vi "configure filter.vi"(7 "extended id? (F)":bool, 8 "error in (no error)":errorcluster, 9 "to id":u32 format="%x", 10 "from id":u32 format="%x", 11 "channel":u16 format="%x") -> (0 "error out":errorcluster)   [LabVIEW 2024, in "atsj peakcan basic.lvlib"]
doc: "Configures the reception filter for a PeakCAN <b>channel</b>."
uses:
  atsj peakcan basic.lvlib
  support/x64/PCANBasic.dll
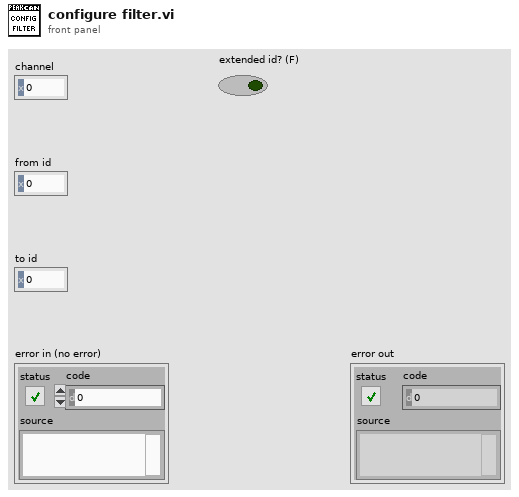
[diagram p1: front panel]
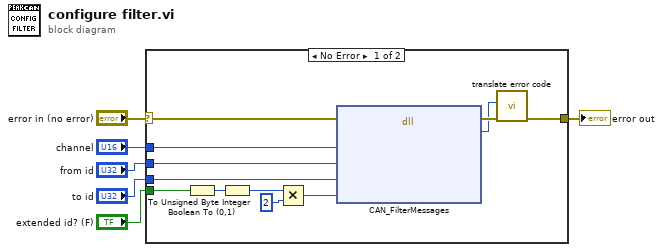
[diagram p0: block diagram]
diagram:
  n1 = case shown="No Error" "error in (no error)" {
    selector: "error in (no error)" -> [w17 w19]
    tunnel: [w8 w19] -> w5
    tunnel: "channel" -> [w18 _]
    tunnel: "extended id? (F)" -> [w16 _]
    tunnel: "from id" -> [w11 _]
    tunnel: "to id" -> [w10 _]
    frame No Error {
      n2 = Boolean To (0,1)(Boolean=w16) -> (0, 1=w15:i16)
      n3 = To Unsigned Byte Integer(number=w15) -> (unsigned 8bit integer=w14:u8)
      n4 = Multiply(x=w14, y=u8 2) -> (x*y=w12:u8)
      n5 = dll-call lib="C:/atsj/plateau/atsj-peakcan-basic-for-labview/src/support/x64/PCANBasic.dll" fn="CAN_FilterMessages" ("configure filter")(error in=w17, "Channel"=w18, "FromID"=w11, "ToID"=w10, "Mode"=w12) -> (error out=w9:errorcluster, "Status"=w7:u32)  [unwired: 6 in, 1 out]
      n6 = call "translate error code.vi"("error in (no error)"=w9, "error code"=w7) -> ("error out"=w8:errorcluster)  [unwired: 9 in]
    }
    frame Error {
    }
  }
  "error out" <- w5
